vi "EventDataToShotNumber.vi"(11 "EventDataIn":u8[](array[numeric])) -> (3 "ShotNumberOut":i32)   [LabVIEW 2011]
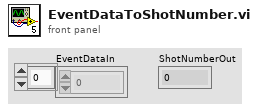
[diagram p1: front panel]
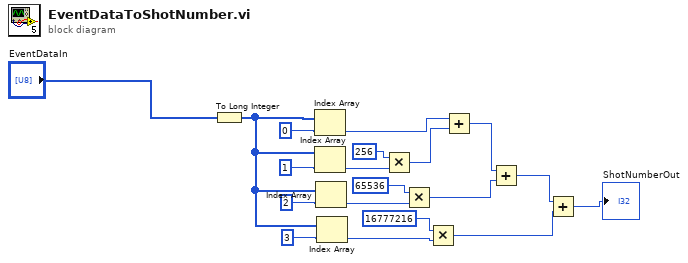
[diagram p0: block diagram]
diagram:
  n1 = To Long Integer(number="EventDataIn") -> (32bit integer=w6:i32[])
  n2 = Index Array(array=w6, index=0) -> (element=w9:i32)
  n3 = Index Array(array=w6, index=1) -> (element=w8:i32)
  n4 = Index Array(array=w6, index=2) -> (element=w11:i32)
  n5 = Index Array(array=w6, index=3) -> (element=w15:i32)
  n6 = Multiply(x=256, y=w8) -> (x*y=w10:i32)
  n7 = Multiply(x=65536, y=w11) -> (x*y=w14:i32)
  n8 = Multiply(x=16777216, y=w15) -> (x*y=w17:i32)
  n9 = Add(x=w9, y=w10) -> (x+y=w13:i32)
  n10 = Add(x=w13, y=w14) -> (x+y=w18:i32)
  n11 = Add(x=w18, y=w17) -> (x+y=→"ShotNumberOut":i32)
